vi "IMAQ Transparency Merge.vi"() -> ()   [LabVIEW 2018]
doc: "Demonstrates how to overlay a image with a transparent image\n\nLabVIEW only recognizes binary states for pixels: full transparency or full opaqueness\nKB 3T9924OA: Reading 32-Bit PNG Files with LabVIEW\nhttp://digital.ni.com/public.nsf/allkb/EEDD9D6EAB559B73862570F200584773?OpenDocument"
panel:
  in  "position":cluster{"X":i32, "Y":i32}={"X"=300, "Y"=100}
  out "Image with Overlay":T1(plugin-control)
  # "Overview: Demonstrates how to overlay a image with a transparent image\nRequirements: LabVIEW 2012 Base Development System (or compatible)\n                             Vision Development Module 2012 (or compatible)\nInstructions: \n1. Select whether the transparency of the overlay image shall be preserved\n2. Run the VI"
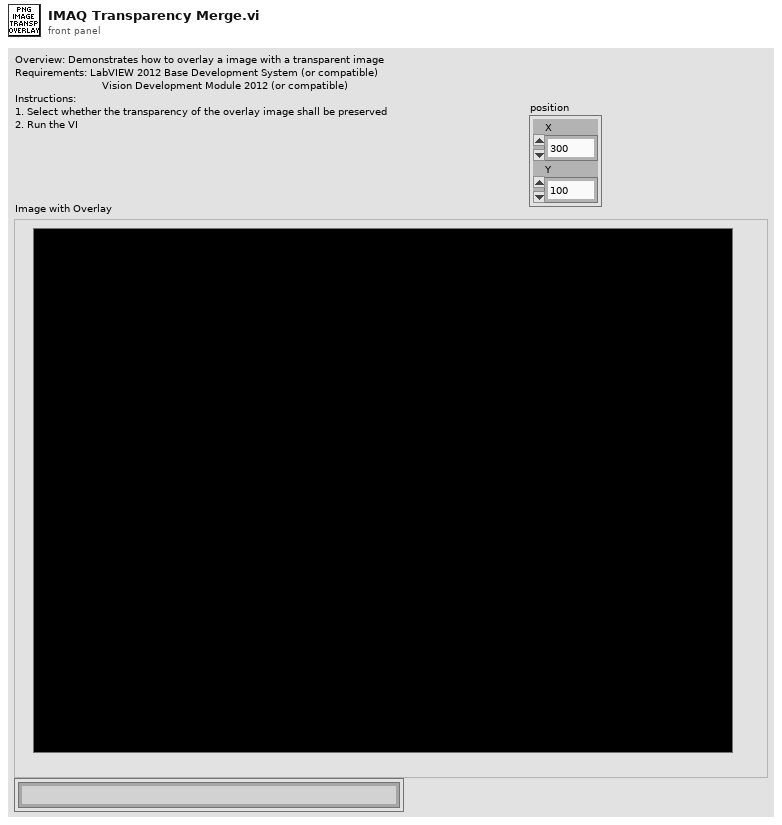
[diagram p1: front panel]
types:
  T1 = typedef "IMAQ Image.ctl" = refnum<image>
  T2 = typedef "Image Type" = u32
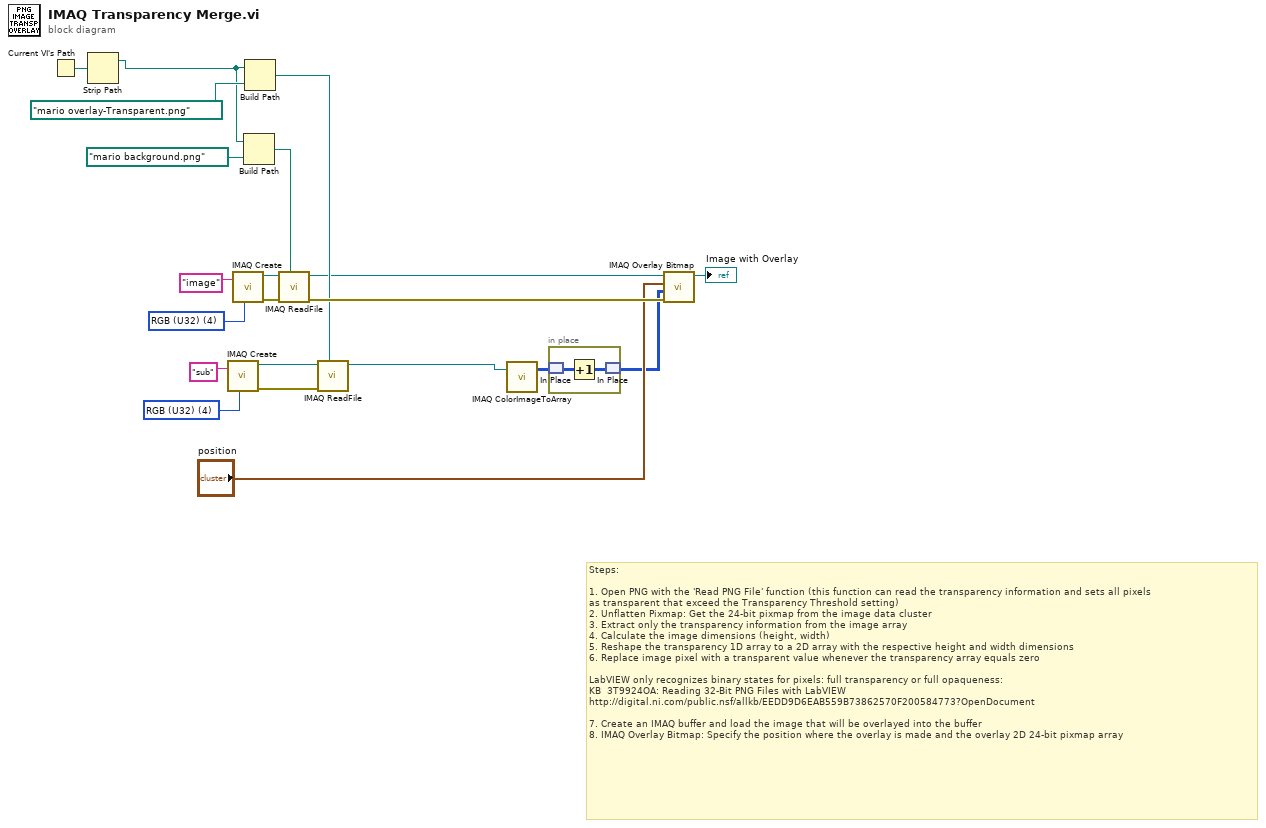
[diagram p0: block diagram]
diagram:
  w8 = T2 4 items=["Grayscale (U8)", "Grayscale (I16)", "Grayscale (SGL)", "Complex (CSG)", "RGB (U32)", "HSL (U32)", "RGB (U64)", "Grayscale (U16)"] ("Image Type")
  w20 = T2 4 items=["Grayscale (U8)", "Grayscale (I16)", "Grayscale (SGL)", "Complex (CSG)", "RGB (U32)", "HSL (U32)", "RGB (U64)", "Grayscale (U16)"] ("Image Type")
  # "Steps:\n\n1. Open PNG with the 'Read PNG File' function (this function can read the transparency information and sets all pixels\nas transparent that exceed the Transparency Threshold setting)\n2. Unflatten Pixmap: Get the 24-bit pixmap from the image data cluster\n3. Extract only the transparency information from the image array\n4. Calculate the image dimensions (height, width)\n5. Reshape the transparency 1D array to a 2D array with the respective height and width dimensions\n6. Replace image pixel with a transparent value whenever the transparency array equals zero\n\nLabVIEW only recognizes binary states for pixels: full transparency or full opaqueness:\nKB  3T9924OA: Reading 32-Bit PNG Files with LabVIEW\nhttp://digital.ni.com/public.nsf/allkb/EEDD9D6EAB559B73862570F200584773?OpenDocument\n\n7. Create an IMAQ buffer and load the image that will be overlayed into the buffer\n8. IMAQ Overlay Bitmap: Specify the position where the overlay is made and the overlay 2D 24-bit pixmap array"
  n1 = Current VI's Path() -> (path=w14:path)
  n2 = Strip Path(path=w14) -> (stripped path=w4:path)  [unwired: 1 out]
  n3 = call "IMAQ Create"("Image Name"="sub", "Image Type"=w8) -> ("New Image"=w10:T1, "error out"=w7:errorcluster)  [unwired: 3 in]
  n4 = call "IMAQ Create"("Image Name"="image", "Image Type"=w20) -> ("New Image"=w18:T1, "error out"=w21:errorcluster)  [unwired: 3 in]
  n5 = Build Path(base path=w4, name or relative path=path "mario background.png" ("stripped path")) -> (appended path=w11:path)
  n6 = Build Path(base path=w4, name or relative path=path "mario overlay-Transparent.png" ("stripped path")) -> (appended path=w5:path)
  n7 = call "IMAQ ReadFile"("File Path"=w11, "error in (no error)"=w21, "Image"=w18) -> ("error out"=w16:errorcluster, "Image Out"=w2:T1)  [unwired: 4 in, 3 out]
  n8 = call "IMAQ ReadFile"("File Path"=w5, "error in (no error)"=w7, "Image"=w10) -> ("Image Out"=w3:T1)  [unwired: 4 in, 4 out]
  n9 = call "IMAQ ColorImageToArray"("Image"=w3) -> ("Image Pixels (U32)"=w6:u32[][])  [unwired: 3 in, 2 out]
  n10 = in-place {
    n11 = in-place-match #1(w6) -> (w23:u32[][])
    n12 = Increment(x=w23) -> (x+1=w22:u32[][])
    n13 = in-place-match #1(w22) -> (w1:u32[][])
  }
  n14 = call "IMAQ Overlay Bitmap"("error in (no error)"=w16, "Bitmap"=w1, "Top Left Point"="position", "Image"=w2) -> ("Image Out"=→"Image with Overlay":T1)  [unwired: 6 in, 1 out]
